vi "From Serial Form.vi"(6 "Serial Version":T1, 10 "Deserializer in":refnum<class "Deserializer.lvclass">, 11 "ArrayIterator in":refnum<class "ArrayIterator.lvclass">) -> (0 "error out":errorcluster, 2 "Deserializer out":refnum<class "Deserializer.lvclass">, 3 "ArrayIterator out":refnum<class "ArrayIterator.lvclass">)   [LabVIEW 2015, in "ArrayIterator.lvclass"]
uses:
  ArrayIterator.lvclass
  <vilib>/NI/AQ Character Lineator/Deserializer/Deserializer.lvclass
  <vilib>/NI/AQ Character Lineator/Serialization Common/Serial Version.ctl
  Interface/Iterator.lvclass
  <vilib>/NI/AQ Character Lineator/Serialization Common/Serialization Common.lvlib
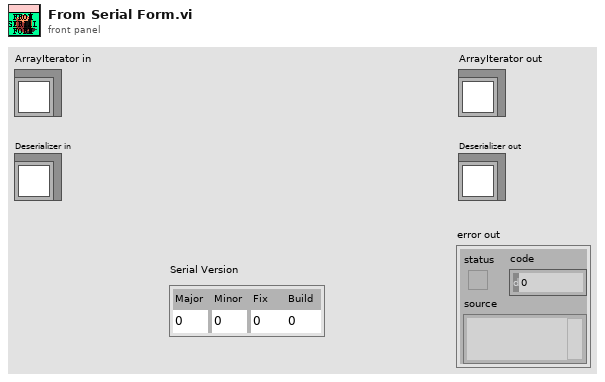
[diagram p1: front panel]
types:
  T1 = typedef "Serialization Common.lvlib/Serial Version.ctl" = cluster{"Major":u16, "Minor":u16, "Fix":u16, "Build":u16}
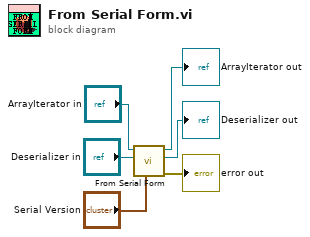
[diagram p0: block diagram]
diagram:
  n1 = call-parent "From Serial Form.vi"("Serial Version"="Serial Version", "Deserializer in"="Deserializer in", "Iterator in"="ArrayIterator in") -> ("error out"=→"error out":errorcluster, "Deserializer out"=→"Deserializer out":refnum<class "Deserializer.lvclass">, "Iterator out"=→"ArrayIterator out":refnum<class "ArrayIterator.lvclass">)  [unwired: 6 in]
